vi "Process Data.vi"(7 "AdasLvTemplate in":refnum<class "AdasLvTemplate.lvclass">, 8 "error in":errorcluster, 11 "Node in":refnum<class "BTSTemplateTest.lvclass">) -> (0 "error out":errorcluster, 3 "Node out":refnum<class "BTSTemplateTest.lvclass">, 5 "AdasLvTemplate out":refnum<class "AdasLvTemplate.lvclass">)   [LabVIEW 2023, in "BTSTemplateTest.lvlib" / "BTSTemplateTest.lvclass"]
uses:
  BTSTemplateTest.lvclass
  <vilib>/ADAS Replay HIL/ADAS Plugin Utilities/AdasLvTemplate/AdasLvTemplate.lvclass
  BTSTemplateTest.lvclass/BTSTemplateTest.ctl
  <vilib>/BTS Capabilities/Cycler/Cycler.lvclass/Cycler.ctl
  <vilib>/BTS Capabilities/Cycler/Read Enable Output Command (Array).vi
  <vilib>/BTS Capabilities/Cycler/Write Voltage Actual (Single).vi
  <vilib>/ADAS Replay HIL/Channels/Tag Wrapper/Read Channel.vi
  <vilib>/ADAS Replay HIL/Channels/Tag Wrapper/Polymorphic/Read Channel (Boolean).vi
  <vilib>/BTS Capabilities/Cycler/Read Enable Output Command (Array).vi/28ca3c79-95f5-44c6-ac38-ea14683abb8a.vi
  <vilib>/ADAS Replay HIL/Channels/Tag Wrapper/Write Channel.vi
  <vilib>/ADAS Replay HIL/Channels/Tag Wrapper/Polymorphic/Write Channel (Double).vi
  <vilib>/ADAS Replay HIL/Channels/Tag Wrapper/Polymorphic/Read Channel (Boolean).vi/b2f764de-0c1e-4784-a155-687fc995a684.vi
  <vilib>/ADAS Replay HIL/Channels/Tag Wrapper/Polymorphic/Write Channel (Double).vi/cccb8e89-591f-4bb4-9d4e-ae06ba1f5498.vi
  <vilib>/ADAS Replay HIL/Channels/Tag Wrapper/Polymorphic/Read Channel (Boolean).vi/b2f764de-0c1e-4784-a155-687fc995a684.vi/c28b0ead-42ad-4072-80a2-aca7f2bd7ce3.vi
  <vilib>/ADAS Replay HIL/Channels/Tag Wrapper/Polymorphic/Read Channel (Boolean).vi/b2f764de-0c1e-4784-a155-687fc995a684.vi/219d0231-d98b-4193-b5cc-84f90e3c9091.vi
  <vilib>/ADAS Replay HIL/Channels/Tag Wrapper/Polymorphic/Write Channel (Double).vi/cccb8e89-591f-4bb4-9d4e-ae06ba1f5498.vi/4bc1c15b-36ab-481f-b8dd-c64075ce723a.vi
  <vilib>/ADAS Replay HIL/Channels/Tag Wrapper/Polymorphic/Write Channel (Double).vi/cccb8e89-591f-4bb4-9d4e-ae06ba1f5498.vi/d83cb72b-7713-41fc-a3d1-682de79cf574.vi
  <vilib>/BTS Capabilities/Cycler/Cycler.lvclass
  <vilib>/BTS Capabilities/Cycler/Write Current Actual (Single).vi
  <vilib>/BTS Capabilities/Cycler/Write Power Actual (Single).vi
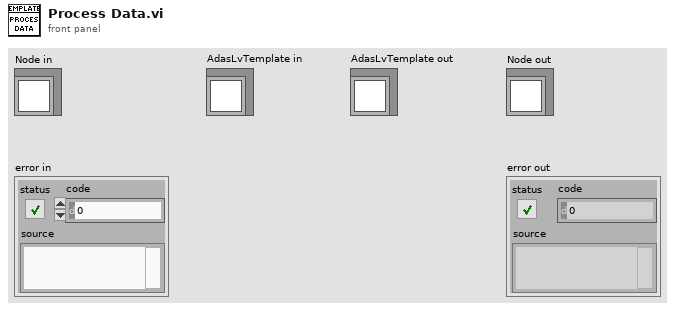
[diagram p1: front panel]
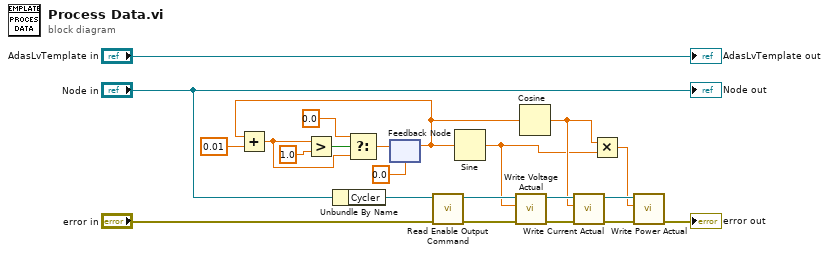
[diagram p0: block diagram]
diagram:
  n1 = Unbundle By Name("Node in") -> ("Cycler"=w20:refnum<class "Cycler.lvclass">)
  n2 = feedback #1(0.0) -> (w15:dbl)
  n3 = Add(x=w15, y=0.01) -> (x+y=w9:dbl)
  n4 = Greater?(x=w9, y=1.0) -> (0:w12:bool)
  n5 = Select(t=0.0 ("f"), s=w12, f=w9) -> (s? t:f=w13:dbl)
  n6 = feedback-in #1(w13) -> ()
  n7 = call-poly <vilib>:"Read Enable Output Command.vi"("error in"="error in", "Cycler in"=w20) -> ("error out"=w18:errorcluster, "Cycler out"=w19:refnum<class "Cycler.lvclass">)  [unwired: 6 in, 2 out]
  n8 = Sine(x=w15) -> (sin(x)=w2:dbl)
  n9 = call-poly <vilib>:"Write Voltage Actual.vi"("error in"=w18, "Voltage"=w2, "Cycler in"=w19) -> ("error out"=w6:errorcluster, "Cycler out"=w7:refnum<class "Cycler.lvclass">)  [unwired: 7 in]
  n10 = Cosine(x=w15) -> (cos(x)=w3:dbl)
  n11 = call-poly <vilib>:"Write Current Actual.vi"("error in"=w6, "Current"=w3, "Cycler in"=w7) -> ("error out"=w4:errorcluster, "Cycler out"=w5:refnum<class "Cycler.lvclass">)  [unwired: 7 in]
  n12 = Multiply(x=w3, y=w2) -> (x*y=w1:dbl)
  n13 = call-poly <vilib>:"Write Power Actual.vi"("error in"=w4, "Power"=w1, "Cycler in"=w5) -> ("error out"=→"error out":errorcluster)  [unwired: 7 in, 1 out]
  "Node out" <- "Node in"
  "AdasLvTemplate out" <- "AdasLvTemplate in"
